vi "ResizeVertexList.vi"(5 "size":i32, 9 "DAG in":refnum<class "DAG.lvclass">) -> (3 "DAG out":refnum<class "DAG.lvclass">)   [LabVIEW 2014, in "DAG.lvclass"]
uses:
  DAG.lvclass
  DAG.lvclass/DAG.ctl
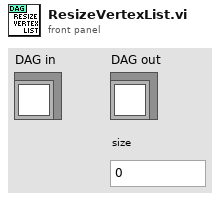
[diagram p1: front panel]
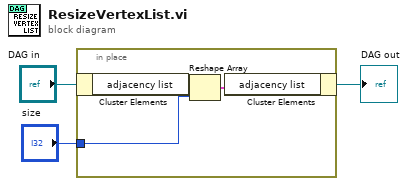
[diagram p0: block diagram]
diagram:
  n1 = in-place {
    in-place-border: "size" -> [w4]
    n2 = in-place-cluster #1("DAG in") -> ("adjacency list"=w6:cluster{"edge list":i32[]}[])
    n3 = Reshape Array(w6, w4) -> (w5:cluster{"edge list":i32[]}[])
    n4 = in-place-cluster #1("adjacency list"=w5) -> (→"DAG out":refnum<class "DAG.lvclass">)
  }
